vi "READDD.vi"(8 "error in":errorcluster) -> (0 "error out":errorcluster, 3 "task out":refnum<k21>)   [LabVIEW 2020]
uses:
  <vilib>/DAQmx/create/channels.llb/DAQmx Create Channel (AO-Voltage-Basic).vi
  <vilib>/DAQmx/configure/timing.llb/DAQmx Timing (Sample Clock).vi
  <resource>/objmgr/daqmx.rc
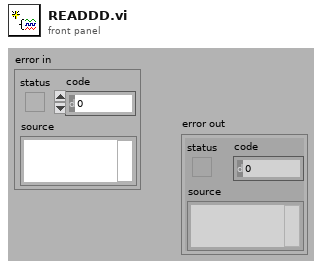
[diagram p1: front panel]
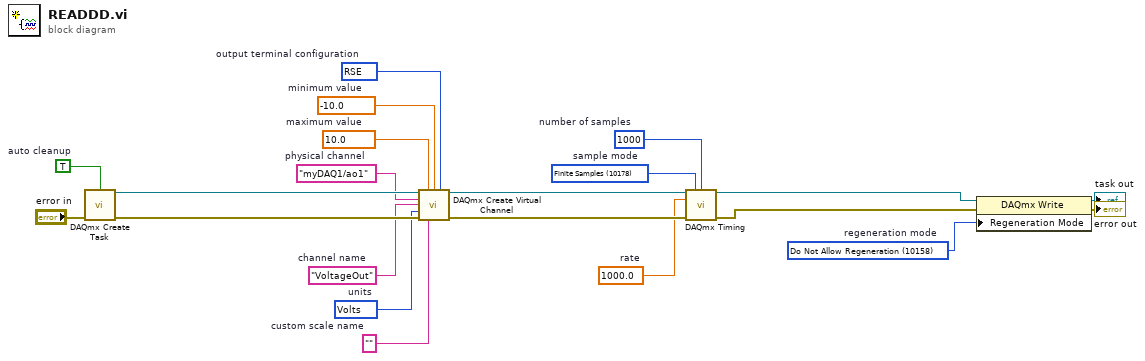
[diagram p0: block diagram]
diagram:
  w1 = 10158 items=["Allow Regeneration"=10097, "Do Not Allow Regeneration"=10158]  # regeneration mode
  w5 = 10178 items=["Finite Samples"=10178, "Continuous Samples"=10123, "Hardware Timed Single Point"=12522]  # sample mode
  w6 = 1000  # number of samples
  w7 = 1000.0  # rate
  w10 = 10083 items=["Default"=-1, "RSE"=10083, "Differential"=10106, "Pseudodifferential"=12529]  # output terminal configuration
  w11 = 10348 items=["Volts"=10348, "From Custom Scale"=10065]  # units
  w12 = "VoltageOut"  # channel name
  w14 = ""  # custom scale name
  w15 = -10.0  # minimum value
  w16 = 10.0  # maximum value
  w17 = "myDAQ1/ao1"  # physical channel
  w19 = TRUE  # auto cleanup
  n1 = call <vilib>:"DAQmx Create Task.vi"("auto cleanup"=w19, "error in"="error in") -> ("task out"=w18:refnum<k21>, "error out"=w20:errorcluster)  [unwired: 12 in]
  n2 = call-poly <vilib>:"DAQmx Create Virtual Channel.vi"("task in"=w18, "maximum value"=w16, "minimum value"=w15, "output terminal configuration"=w10, "physical channels"=w17, "name to assign"=w12, "units"=w11, "error in"=w20, "custom scale name"=w14) -> ("task out"=w8:refnum<k21>, "error out"=w13:errorcluster)  [unwired: 5 in]
  n3 = call-poly <vilib>:"DAQmx Timing.vi"("task/channels in"=w8, "sample mode"=w5, "samples per channel"=w6, "rate"=w7, "error in"=w13) -> ("task out"=w4:refnum<k21>, "error out"=w9:errorcluster)  [unwired: 9 in]
  n4 = property class="DAQmx Write"(reference=w4, error in=w9, "Regeneration Mode"=w1) -> (reference out=→"task out":refnum<k21>, error out=→"error out":errorcluster)
